vi "Database_Remove_Patient.vi"(11 "Patient_ID":string) -> (3 "Patient List":string[][](array[string]))   [LabVIEW 2013, in "Medimatic.lvlib"]
uses:
  Medimatic.lvlib
  Globals/DataPathGlobalVariable.vi
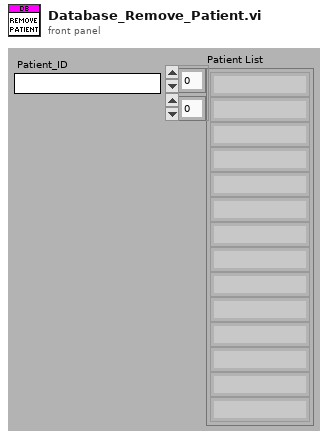
[diagram p1: front panel]
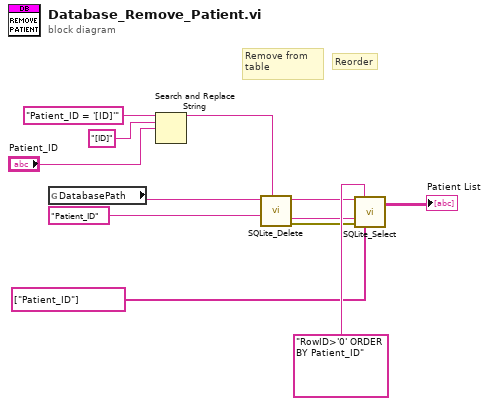
[diagram p0: block diagram]
diagram:
  # "Reorder"
  # "Remove from table"
  n1 = global read "DataPathGlobalVariable.vi" "DatabasePath"() -> (w11:string)
  n2 = Search and Replace String(input string="Patient_ID = '[ID]'" ("string"), search string="[ID]", replace string="Patient_ID") -> (result string=w1:string)  [unwired: 5 in, 3 out]
  n3 = call <userlib>:"SQLite_Delete.vi"("Where Clause"=w1, "Table Name"="Patient_ID", "DB Path"=w11) -> ("error out"=w8:errorcluster, "Table Name Out"=w7:string, "DB Path Out"=w9:string)  [unwired: 4 in]
  n4 = call <userlib>:"SQLite_Select.vi"("DB Path"=w9, "Where Clause"="RowID>'0' ORDER BY Patient_ID", "Table Name"=w7, "error in (no error)"=w8, "Columns"=string[] ["Patient_ID"]) -> ("Results"=→"Patient List":string[][])  [unwired: 7 in, 3 out]
